vi "set_ENA_statuses.vi"(8 "error in (no error)":errorcluster caption="错误输入（无错误）", 10 "ENA statuses":bool[](array[boolean]), 11 "MotorSystem 输入":refnum<class "MotorSystem.lvclass">) -> (0 "error out":errorcluster caption="错误输出", 3 "MotorSystem 输出":refnum<class "MotorSystem.lvclass">)   [LabVIEW 2016, in "MotionControl.lvlib" / "MotorSystem.lvclass"]
uses:
  <userlib>/MotionControl/MotorSystem/MotorSystem.lvclass
  <userlib>/MotionControl/MotorSystem/MotorSystem.lvclass/MotorSystem.ctl
  <userlib>/MotionControl/OneMotion/OneMotion.lvclass
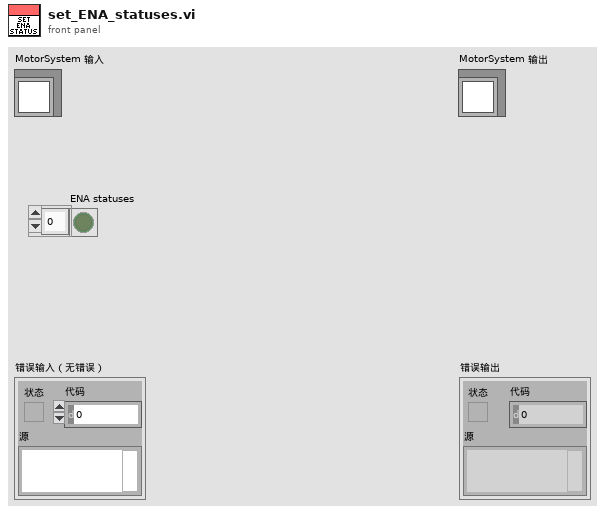
[diagram p1: front panel]
types:
  T1 = typedef "MotionControl.lvlib/MotorSystem.lvclass/MotionCluster.ctl" = cluster{"OneMotion.lvclass":refnum<class "OneMotion.lvclass">, "connected?":bool, "default enabled?":bool, "enabled?":bool}
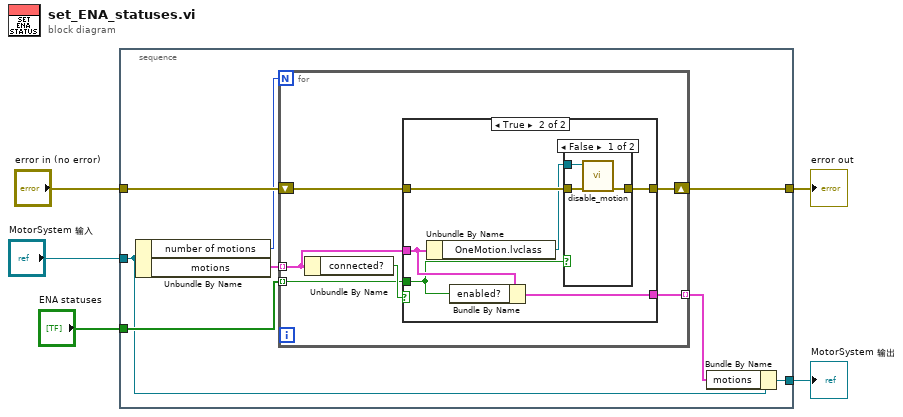
[diagram p0: block diagram]
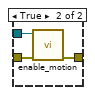
[diagram p3: hidden frame]
diagram:
  n1 = stacked-sequence {
    tunnel: [w11] -> w5
    tunnel: [w7] -> w3
    tunnel: "MotorSystem 输入" -> [w8]
    tunnel: "error in (no error)" -> [w12]
    tunnel: "ENA statuses" -> [w10]
    frame #0 {
      n2 = Unbundle By Name(w8) -> ("number of motions"=w6:i32, "motions"=w13:T1[])
      n3 = for {
        N: w6 -> [_]
        tunnel: w13 -> [w17] mode=indexing
        shift-right: [w18] -> w11
        shift-left: w12 -> [w19]
        tunnel: w10 -> [w15] mode=indexing
        tunnel: [w14] -> w9 mode=indexing
        n4 = Unbundle By Name(w17) -> ("connected?"=w16:bool)
        n5 = case shown="True" w16 {
          tunnel: w17 -> [w20 w24]
          tunnel: w19 -> [w21 w27]
          tunnel: [w21 w25] -> w18
          tunnel: w15 -> [_ w23]
          tunnel: [w20 w22] -> w14
          frame False {
          }
          frame True {
            n6 = Unbundle By Name(w24) -> ("OneMotion.lvclass"=w26:refnum<class "OneMotion.lvclass">)
            n7 = Bundle By Name(cluster=w24, "enabled?"=w23) -> (w22:T1)
            n8 = case shown="False" w23 {
              tunnel: w27 -> [w29 w33]
              tunnel: w26 -> [w30 w32]
              tunnel: [w28 w31] -> w25
              frame False {
                n9 = call <userlib>:"disable_motion.vi"("error in (no error)"=w29, "OneMotion 输入"=w30) -> ("error out"=w28:errorcluster)  [unwired: 8 in, 1 out]
              }
              frame True {
                n10 = call <userlib>:"enable_motion.vi"("error in (no error)"=w33, "OneMotion 输入"=w32) -> ("error out"=w31:errorcluster)  [unwired: 8 in, 1 out]
              }
            }
          }
        }
      }
      n11 = Bundle By Name(cluster=w8, "motions"=w9) -> (w7:refnum<class "MotorSystem.lvclass">)
    }
  }
  "error out" <- w5
  "MotorSystem 输出" <- w3
